vi "Serialize as XML.vi"(8 "error in (no error)":errorcluster, 11 "Element Array in":refnum<class "Element Array.lvclass">) -> (0 "error out":errorcluster, 2 "XML Fragment":string, 3 "Element Array out":refnum<class "Element Array.lvclass">)   [LabVIEW 2023, in "VILab.lvlib" / "Element Array.lvclass"]
uses:
  Element Array.lvclass
  Element Array.lvclass/Element Array.ctl
  Attribute.lvclass
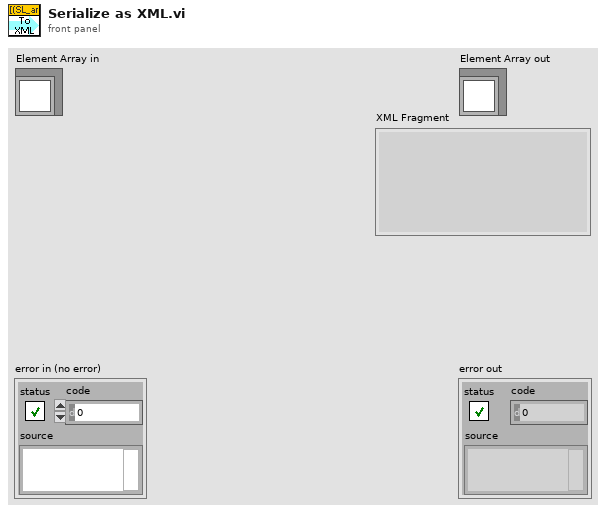
[diagram p1: front panel]
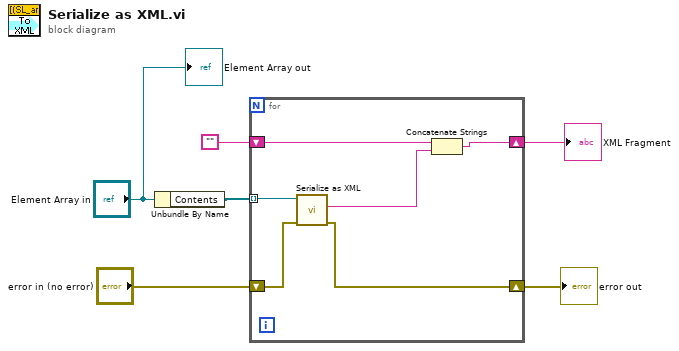
[diagram p0: block diagram]
diagram:
  n1 = Unbundle By Name("Element Array in") -> ("Contents"=w6:refnum<class "Attribute.lvclass">[])
  n2 = for {
    tunnel: w6 -> [w11] mode=indexing
    shift-right: [w7] -> w3
    shift-left: "" -> [w12]
    shift-right: [w9] -> w2
    shift-left: "error in (no error)" -> [w10]
    n3 = call-dynamic "Serialize as XML.vi"("error in (no error)"=w10, "Attribute in"=w11) -> ("error out"=w9:errorcluster, "XML Fragment"=w8:string)  [unwired: 7 in, 1 out]
    n4 = Concatenate Strings(w12, w8) -> (w7:string)
  }
  "error out" <- w2
  "XML Fragment" <- w3
  "Element Array out" <- "Element Array in"
